vi "Digital Pattern Page - Multi FPGA.vi"(8 "error in (no error)":errorcluster, 11 "Node Ptr":T1 format="%.0x") -> (0 "error out":errorcluster)   [LabVIEW 2015, in "Engine Simulation Toolkit System Explorer.lvlib"]
uses:
  Engine Simulation Toolkit System Explorer.lvlib
  <vilib>/NI Veristand/Custom Device API/Custom Device Item Ref.ctl
  Shared/Properties.vi
  <vilib>/NI Veristand/Custom Device API/Get Item Property (String).vi
  <vilib>/NI Veristand/Custom Device API/Custom Device API.lvlib
  Shared/Engine Simulation Toolkit Shared.lvlib
panel:
  out "Name in bitfile":string
  in  "Name":string
  in  "Header":cluster{"Section Name":string}={"Section Name"="Digital Pattern"}
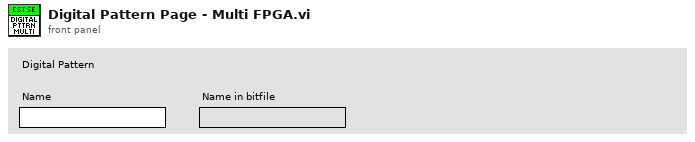
[diagram p1: front panel]
types:
  T1 = typedef "Custom Device API.lvlib/Custom Device Item Ref.ctl" = u64
  T2 = typedef "Custom Device API.lvlib/Custom Device Item Info.ctl" = cluster{"Name":string, "Is Channel":bool, "GUID":string, "Is Waveform":bool}
  T3 = typedef "Custom Device API.lvlib/Custom Device Commands.ctl" = enum16{"Default", "Item renamed", "Shutdown", "Dynamic button pressed"}
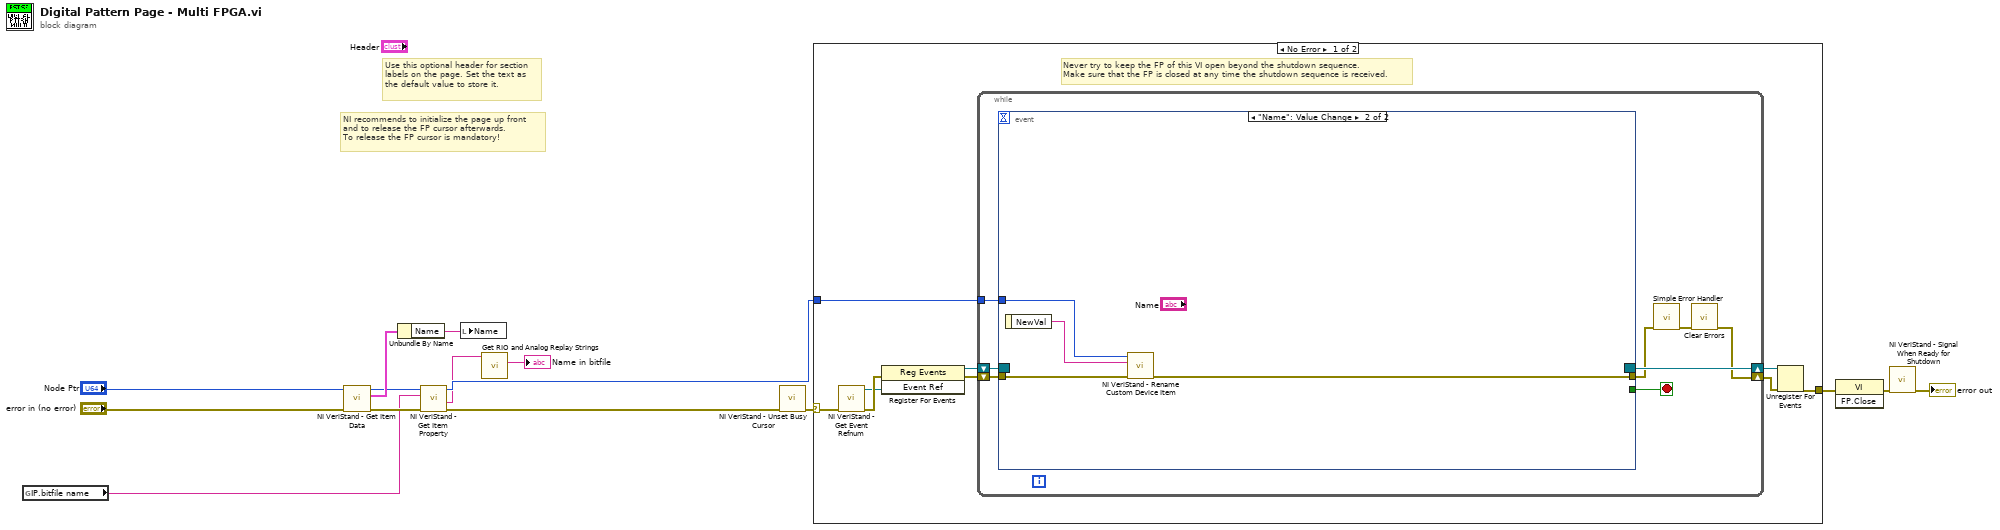
[diagram p0: block diagram]
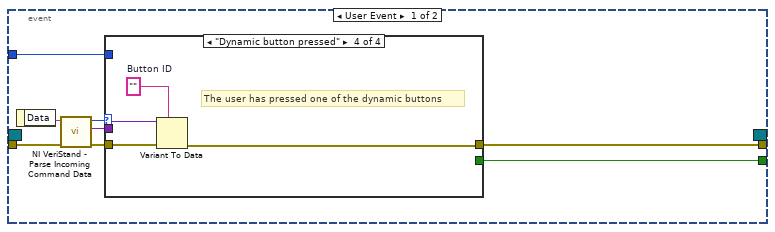
[diagram p2: hidden frame]
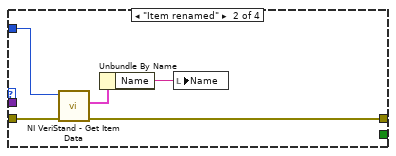
[diagram p4: hidden frame]
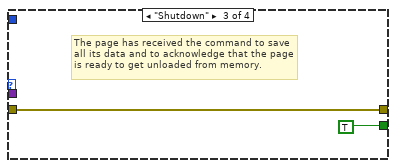
[diagram p5: hidden frame]
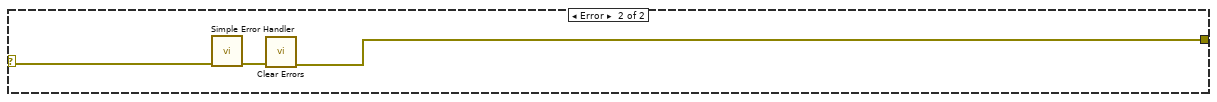
[diagram p6: hidden frame]
diagram:
  # "Use this optional header for section labels on the page. Set the text as the default value to store it."
  # "NI recommends to initialize the page up front\nand to release the FP cursor afterwards.\nTo release the FP cursor is mandatory!"
  n1 = global read "Properties.vi" "IP.bitfile name"() -> (w3:string)
  n2 = call <vilib>:"NI VeriStand - Get Item Data.vi"("error in (no error)"="error in (no error)", "Item Ref in"="Node Ptr") -> ("error out"=w9:errorcluster, "Item Info"=w8:T2, "Item Ref out"=w5:T1)  [unwired: 6 in, 1 out]
  n3 = Unbundle By Name(w8) -> ("Name"=w7:string)
  n4 = call-poly <vilib>:"NI VeriStand - Get Item Property.vi"("error in (no error)"=w9, "Property Name"=w3, "Item Ref in"=w5) -> ("error out"=w6:errorcluster, "Value"=w2:string, "Item Ref out"=w4:T1)  [unwired: 5 in, 1 out]
  n5 = local write "Name"(w7) -> ()
  n6 = call "Get RIO and Analog Replay Strings.vi"("rio/analog replay"=w2) -> ("analog replay"=→"Name in bitfile":string)  [unwired: 9 in, 1 out]
  n7 = call <vilib>:"NI VeriStand - Unset Busy Cursor.vi"("error in (no error)"=w6) -> ("error out"=w11:errorcluster)  [unwired: 10 out]
  n8 = case shown="No Error" w11 {
    selector: w11 -> [w16 w59]
    tunnel: [w21 w57] -> w15
    tunnel: w4 -> [w17 _]
    frame No Error {
      # "Never try to keep the FP of this VI open beyond the shutdown sequence.\nMake sure that the FP is closed at any time the shutdown sequence is received."
      n9 = call <vilib>:"NI VeriStand - Get Event Refnum.vi"("error in (no error)"=w16) -> ("error out"=w24:errorcluster, "Event Ref"=w20:refnum<user-event>)  [unwired: 9 out]
      n10 = register-events(error in=w24, w20) -> (reference out=w18:refnum<event-registration>, error out=w19:errorcluster)  [unwired: 1 in]
      n11 = while {
        tunnel: w17 -> [w28]
        shift-right: [w25] -> w22
        shift-left: w19 -> [w31]
        shift-right: [w32] -> w23
        shift-left: w18 -> [w30]
        stop <- w29 stop-if-true
        n12 = event shown="[1] \"Name\": Value Change" {
          selector: w30 -> [_ _]
          dyn-events: [_ _] -> w32
          timeout: _ -> [_ _]
          tunnel: w31 -> [w40 w56]
          tunnel: [w36 _] -> w29
          tunnel: [w35 w55] -> w27
          tunnel: w28 -> [w34 w54]
          event User Event {
            n13 = event-data() -> ("Data"=w39:string)  [unwired: 1 out]
            n14 = call <vilib>:"NI VeriStand - Parse Incoming Command Data.vi"("error in (no error)"=w40, "Incoming data"=w39) -> ("error out"=w38:errorcluster, "Outgoing data"=w33:variant, "Action"=w37:T3)  [unwired: 7 out]
            n15 = case shown="\"Dynamic button pressed\"" w37 {
              tunnel: w38 -> [w41 w46 w47 w52]
              tunnel: [_ _ TRUE _] -> w36
              tunnel: [w41 w42 w47 w49] -> w35
              tunnel: w34 -> [_ w45 _ _]
              tunnel: w33 -> [_ _ _ w51]
              frame "Default", Default {
              }
              frame "Item renamed" {
                n16 = call <vilib>:"NI VeriStand - Get Item Data.vi"("error in (no error)"=w46, "Item Ref in"=w45) -> ("error out"=w42:errorcluster, "Item Info"=w43:T2)  [unwired: 6 in, 2 out]
                n17 = Unbundle By Name(w43) -> ("Name"=w44:string)
                n18 = local write "Name"(w44) -> ()
              }
              frame "Shutdown" {
                # "The page has received the command to save all its data and to acknowledge that the page is ready to get unloaded from memory."
              }
              frame "Dynamic button pressed" {
                w50 = ""  # Button ID
                # "The user has pressed one of the dynamic buttons"
                n19 = Variant To Data(error in=w52, type=w50, Variant=w51) -> (error out=w49:errorcluster)  [unwired: 1 out]
              }
            }
          }
          event "Name": Value Change {
            n20 = event-data() -> ("NewVal"=w53:string)  [unwired: 1 out]
            n21 = call <vilib>:"NI VeriStand - Rename Custom Device Item.vi"("error in (no error)"=w56, "New Name"=w53, "Item Ref in"=w54) -> ("error out"=w55:errorcluster)  [unwired: 6 in, 2 out]
          }
        }
        n22 = call <vilib>:"Simple Error Handler.vi"("error in (no error)"=w27) -> ("error out"=w26:errorcluster)  [unwired: 1 in, 7 out]
        n23 = call <vilib>:"Clear Errors.vi"("error in (no error)"=w26) -> ("error out"=w25:errorcluster)  [unwired: 1 in, 5 out]
      }
      n24 = Unregister For Events(event registration refnum=w23, error in=w22) -> (error out=w21:errorcluster)
    }
    frame Error {
      n25 = call <vilib>:"Simple Error Handler.vi"("error in (no error)"=w59) -> ("error out"=w58:errorcluster)  [unwired: 1 in, 7 out]
      n26 = call <vilib>:"Clear Errors.vi"("error in (no error)"=w58) -> ("error out"=w57:errorcluster)  [unwired: 1 in, 5 out]
    }
  }
  n27 = invoke class="VI" method="FP.Close"(error in=w15) -> (error out=w14:errorcluster)  [unwired: 2 in, 2 out]
  n28 = call <vilib>:"NI VeriStand - Signal When Ready for Shutdown.vi"("error in (no error)"=w14) -> ("error out"=→"error out":errorcluster)  [unwired: 10 out]
